vi "Draw Image to Picture (Greyscale with Mask).vi"(7 "Image Draw Offset (Default 0,0)":T2, 8 "error in (no error)":errorcluster, 10 "Greyscale Mask in":T1, 11 "Greyscale Image Source in":T1) -> (0 "error out":errorcluster, 3 "Picture":picture)   [LabVIEW 2020, in "image.lvlib"]
doc: "Draw an image to a LabVIEW Picture with Mask Data to allow for the output picture to be concatinated with other LabVIEW Picture Data."
uses:
  image.lvlib
  Greyscale Image.ctl
  Image Draw Offset.ctl
  9ae995ca-ccda-485c-89ac-02736fde3e8e.vi
  <vilib>/Utility/error.llb/Error Cluster From Error Code.vi
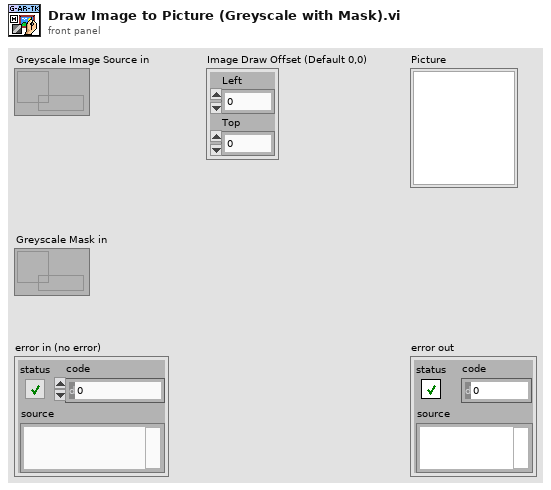
[diagram p1: front panel]
types:
  T1 = typedef "image.lvlib/Greyscale Image.ctl" = refnum<data-value>
  T2 = typedef "image.lvlib/Image Draw Offset.ctl" = cluster{"Left":i16, "Top":i16}
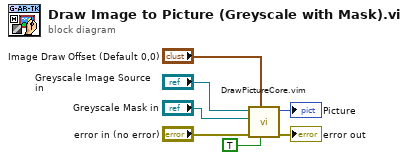
[diagram p0: block diagram]
diagram:
  n1 = call "DrawPictureCore.vim"("HasMask"=TRUE, "Image Draw Offset"="Image Draw Offset (Default 0,0)", "error in (no error)"="error in (no error)", "Image Mask"="Greyscale Mask in", "Image Src"="Greyscale Image Source in") -> ("error out"=→"error out":errorcluster, "Picture"=→"Picture":picture)  [unwired: 5 in]
